vi "Do a Script.vi"() -> ()   [LabVIEW 2012]
panel:
  in  "script":string="--Does a script that uses some of the LuaVIEW\n--functions in the public function registry. This registry\n--is automatically initialized the first time a script is run\n--provided that the \"auto-init registry\" global is set.\n\nprint(\"Hello world\")\nprint(\"The time is \"..format_time(time(),\"%H:%M\"))\nfor i=10,1,-1 do\n    print(i)\n    wait(300) \nend\nprint(\"Lift off!\")\nwait(2000)\ndialog.one_button(\"Launch sequence complete\", \"OK\")\n"
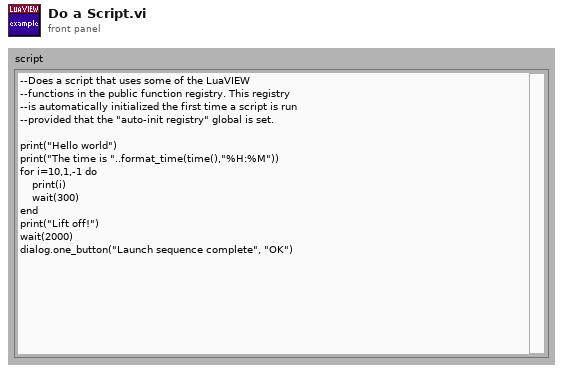
[diagram p1: front panel]
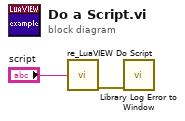
[diagram p0: block diagram]
diagram:
  n1 = call "re_LuaVIEW Do Script.vi"("script string (\"\" == load from file)"="script") -> ("error out"=w2:errorcluster)  [unwired: 14 in]
  n2 = call "Library Log Error to Window.vi"("error in (no error)"=w2) -> ()  [unwired: 13 in, 2 out]
